vi "LaserCal-Init Graphs (I-O).vi"(0 "error in (no error)":errorcluster, 9 "Response":T2, 11 "I-O Data in":T1, 12 "Time Graph":refnum<vi>, 13 "I-O":refnum<vi>) -> (4 "error out":errorcluster, 15 "I-O Data out":T1)   [LabVIEW 2015]
uses:
  Typedefs/LaserCal-Data (I-O).ctl
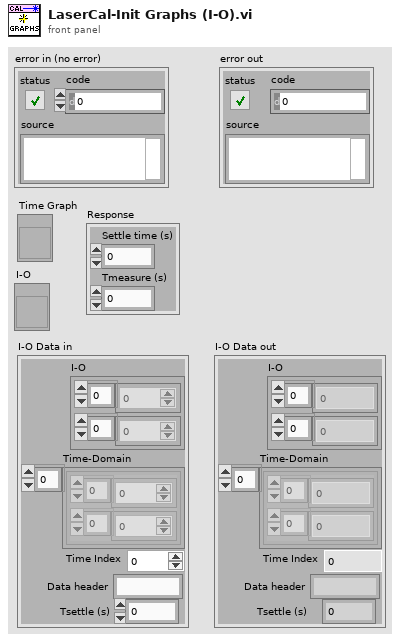
[diagram p1: front panel]
types:
  T1 = typedef "LaserCal-Data (I-O).ctl" = cluster{"I-O":cluster{dbl[], dbl[]}, "Time-Domain":cluster{dbl[], dbl[]}[], "Time Index":i32, "Data header":string, "Tsettle (s)":dbl}
  T2 = cluster{"Settle time (s)":dbl, "Tmeasure (s)":dbl}
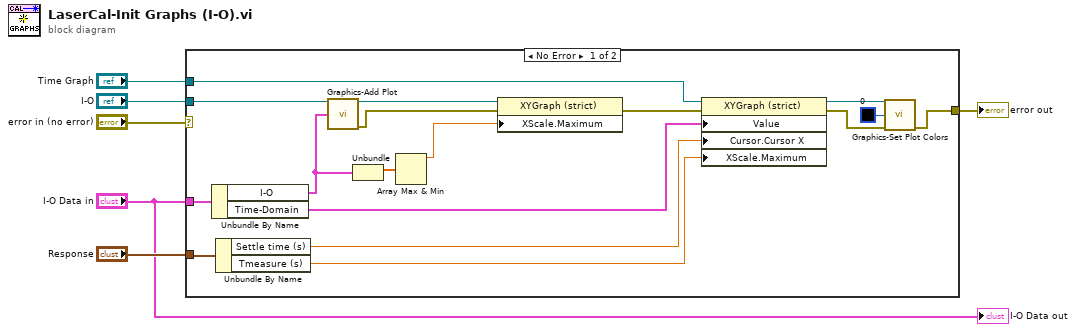
[diagram p0: block diagram]
diagram:
  n1 = case shown="No Error" "error in (no error)" {
    selector: "error in (no error)" -> [_ w24]
    tunnel: [w13 w24] -> w3
    tunnel: "Time Graph" -> [w22 _]
    tunnel: "I-O" -> [w15 _]
    tunnel: "I-O Data in" -> [w23 _]
    tunnel: "Response" -> [w20 _]
    frame No Error {
      n2 = Unbundle By Name(w23) -> ("I-O"=w14:cluster{dbl[], dbl[]}, "Time-Domain"=w21:cluster{dbl[], dbl[]}[])
      n3 = Unbundle By Name(w20) -> ("Settle time (s)"=w19:dbl, "Tmeasure (s)"=w17:dbl)
      n4 = call "Graphics-Add Plot.vi"("XYGraph in"=w15, "XY Data"=w14) -> ("XYGraph out"=w10:refnum<vi>, "error out"=w9:errorcluster)  [unwired: 12 in]
      n5 = Unbundle(w14) -> (w16:dbl[])  [unwired: 1 out]
      n6 = Array Max & Min(array=w16) -> (max value=w8:dbl)  [unwired: 3 out]
      n7 = property class="XYGraph (strict)"(reference=w10, error in=w9, "XScale.Maximum"=w8) -> (error out=w7:errorcluster)  [unwired: 1 out]
      n8 = property class="XYGraph (strict)"(reference=w22, error in=w7, "Value"=w21, "Cursor.Cursor X"=w19, "XScale.Maximum"=w17) -> (reference out=w12:refnum<vi>, error out=w18:errorcluster)
      n9 = call "Graphics-Set Plot Colors.vi"("XY Graph"=w12, "Color Box"=u32 0, "error in (no error)"=w18) -> ("error out"=w13:errorcluster)  [unwired: 12 in]
    }
    frame Error {
    }
  }
  "error out" <- w3
  "I-O Data out" <- "I-O Data in"
